vi "Split Integer.vi"(0 "Input":i32) -> (1 "First half":i32, 2 "Second half":i32)   [LabVIEW 2009, in "IDW.lvlib"]
doc: "Splits the <b>Input</b> value in half, if even. If it is odd, adds the extra one to the <b>First half</b>."
uses:
  IDW.lvlib
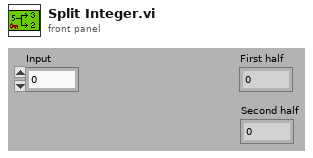
[diagram p1: front panel]
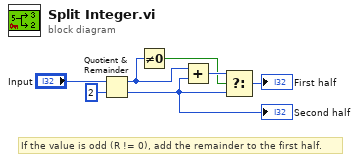
[diagram p0: block diagram]
diagram:
  # "If the value is odd (R != 0), add the remainder to the first half."
  n1 = Quotient & Remainder(x="Input", y=2) -> (x-y*floor(x/y)=w5:i32, floor(x/y)=w4:i32)
  "Second half" <- w4
  n2 = Not Equal To 0?(x=w5) -> (x != 0?=w3:bool)
  n3 = Add(x=w5, y=w4) -> (x+y=w6:i32)
  n4 = Select(t=w6, s=w3, f=w4) -> (s? t:f=→"First half":i32)
